vi "poistion change.vi"(0 "Value":dbl, 1 "方向":u32, 2 "位置":u32) -> (7 "Data":u8[](array[numeric]))   [LabVIEW 2015]
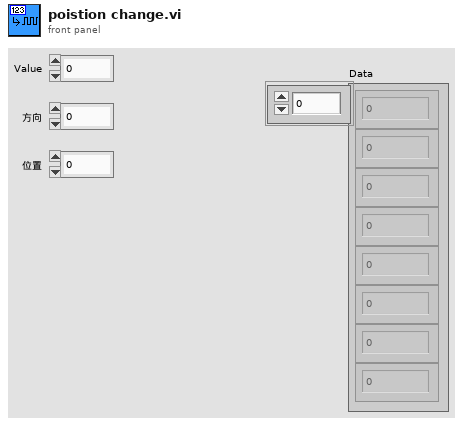
[diagram p1: front panel]
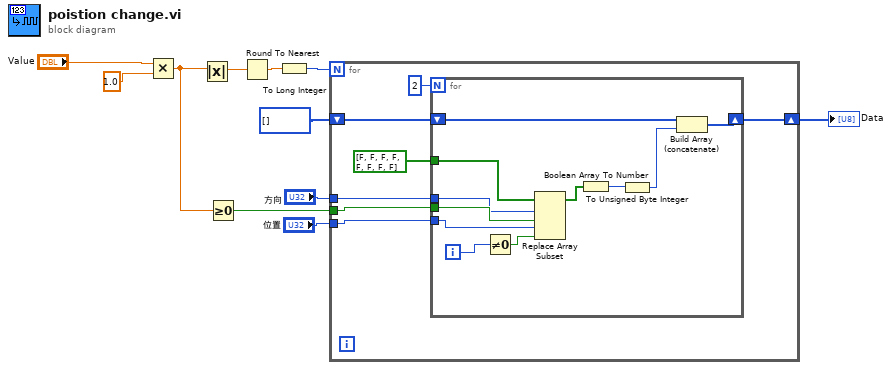
[diagram p0: block diagram]
diagram:
  n1 = Multiply(x="Value", y=1.0) -> (x*y=w2:dbl)
  n2 = Absolute Value(x=w2) -> (abs(x)=w11:dbl)
  n3 = Greater Or Equal To 0?(x=w2) -> (x >= 0?=w8:bool)
  n4 = Round To Nearest(number=w11) -> (nearest integer value=w10:dbl)
  n5 = To Long Integer(number=w10) -> (32bit integer=w9:i32)
  n6 = for {
    N: w9 -> [_]
    shift-right: [w16] -> w6
    shift-left: u8[] [] -> [w18]
    tunnel: w8 -> [w17]
    tunnel: "方向" -> [w13]
    tunnel: "位置" -> [w12]
    n7 = for {
      N: 2 -> [_]
      tunnel: w17 -> [w21]
      shift-right: [w25] -> w16
      shift-left: w18 -> [w28]
      tunnel: bool[] [FALSE, FALSE, FALSE, FALSE, FALSE, FALSE, FALSE, FALSE] -> [w22]
      tunnel: w13 -> [w20]
      tunnel: w12 -> [w19]
      i -> [w24]
      n8 = Not Equal To 0?(x=w24) -> (x != 0?=w23:bool)
      n9 = Replace Array Subset(array=w22, new element #1=w21, index #1=w20, new element #2=w23, index #2=w19) -> (w29:bool[])
      n10 = Boolean Array To Number(Boolean array=w29) -> (number=w27:u32)
      n11 = To Unsigned Byte Integer(number=w27) -> (unsigned 8bit integer=w26:u8)
      n12 = Build Array (concatenate)(w28, w26) -> (w25:u8[])
    }
  }
  "Data" <- w6
